vi "ISO-8601 UTC to Timestamp.vi"(11 "ISO-8601":string) -> (2 "error out":errorcluster, 3 "time stamp":timestamp)   [LabVIEW 2018, in "JSON.lvlib"]
uses:
  JSON.lvlib
  <vilib>/Utility/miscctls.llb/LVDateTimeRec.ctl
  <vilib>/regexp/Match Regular Expression.xnode
panel:
  out "whole match":string
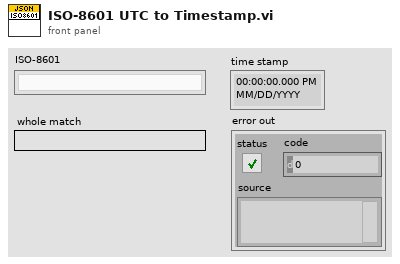
[diagram p1: front panel]
types:
  T1 = typedef "LVDateTimeRec.ctl" = cluster{"fractional second":dbl, "second":i32, "minute":i32, "hour":i32, "day of month":i32, "month":i32, "year":i32, "day of week":i32, "day of year":i32, "DST":i32}
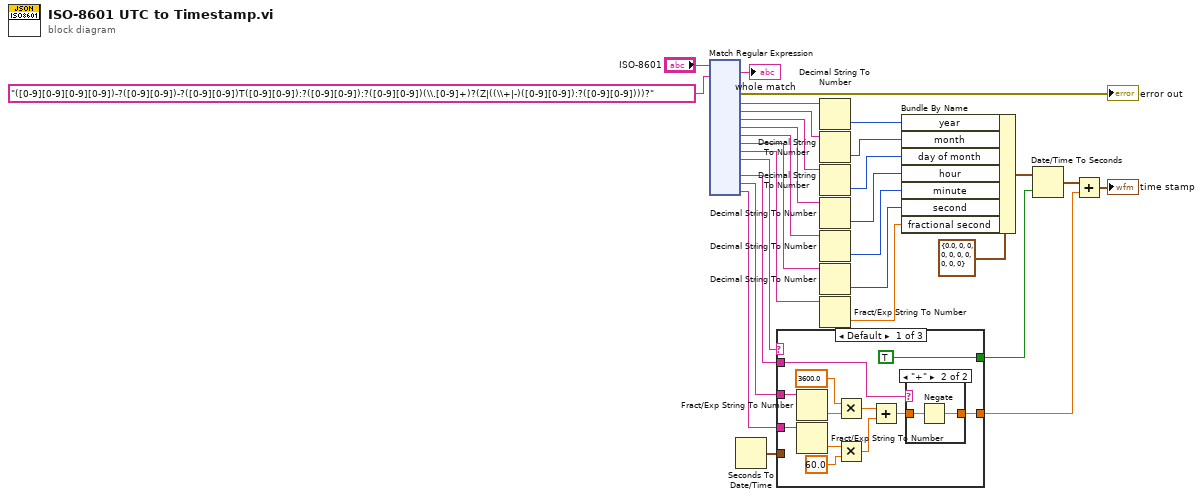
[diagram p0: block diagram]
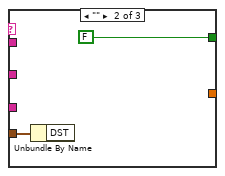
[diagram p3: hidden frame]
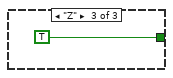
[diagram p4: hidden frame]
diagram:
  n1 = xnode "Match Regular Expression"("input string"="ISO-8601", "regular expression"="([0-9][0-9][0-9][0-9])-?([0-9][0-9])-?([0-9][0-9])T([0-9][0-9]):?([0-9][0-9]):?([0-9][0-9])(\\.[0-9]+)?(Z|((\\+|-)([0-9][0-9]):?([0-9][0-9])))?") -> ("whole match"=→"whole match":string, "error out"=→"error out":errorcluster, "submatch 1"=w27:string, "submatch 2"=w26:string, "submatch 3"=w17:string, "submatch 4"=w16:string, "submatch 5"=w15:string, "submatch 6"=w14:string, "submatch 7"=w13:string, "submatch 8"=w12:string, "submatch 10"=w11:string, "submatch 11"=w10:string, "submatch 12"=w9:string)  [unwired: 4 in, 4 out]
  n2 = Seconds To Date/Time() -> (date time rec=w2:T1)  [unwired: 2 in]
  n3 = case shown="Default" w12 {
    tunnel: w11 -> [w31 _ _]
    tunnel: w10 -> [w40 _ _]
    tunnel: w9 -> [w39 _ _]
    tunnel: [TRUE FALSE TRUE] -> w7
    tunnel: [w30 _ _] -> w4
    tunnel: w2 -> [_ w45 _]
    frame Default {
      n4 = Fract/Exp String To Number(string=w40) -> (number=w38:dbl)  [unwired: 3 in, 1 out]
      n5 = Fract/Exp String To Number(string=w39) -> (number=w37:dbl)  [unwired: 3 in, 1 out]
      n6 = Multiply(x=3600.0 ("y"), y=w38) -> (x*y=w34:dbl)
      n7 = Multiply(x=w37, y=60.0) -> (x*y=w33:dbl)
      n8 = Add(x=w34, y=w33) -> (x+y=w32:dbl)
      n9 = case shown="\"+\"" w31 {
        tunnel: w32 -> [w42 w44]
        tunnel: [w42 w43] -> w30
        frame Default {
        }
        frame "+" {
          n10 = Negate(x=w44) -> (-x=w43:dbl)
        }
      }
    }
    frame "" {
      n11 = Unbundle By Name(w45) -> ()  [unwired: 1 out]
    }
    frame "Z" {
    }
  }
  n12 = Decimal String To Number(string=w27) -> (number=w24:i32)  [unwired: 2 in, 1 out]
  n13 = Decimal String To Number(string=w26) -> (number=w23:i32)  [unwired: 2 in, 1 out]
  n14 = Decimal String To Number(string=w17) -> (number=w22:i32)  [unwired: 2 in, 1 out]
  n15 = Decimal String To Number(string=w16) -> (number=w21:i32)  [unwired: 2 in, 1 out]
  n16 = Decimal String To Number(string=w15) -> (number=w20:i32)  [unwired: 2 in, 1 out]
  n17 = Decimal String To Number(string=w14) -> (number=w19:i32)  [unwired: 2 in, 1 out]
  n18 = Fract/Exp String To Number(string=w13) -> (number=w18:dbl)  [unwired: 3 in, 1 out]
  n19 = Bundle By Name(cluster=T1 {"fractional second"=0.0, "second"=0, "minute"=0, "hour"=0, "day of month"=0, "month"=0, "year"=0, "day of week"=0, "day of year"=0, "DST"=0} ("date time rec"), "year"=w24, "month"=w23, "day of month"=w22, "hour"=w21, "minute"=w20, "second"=w19, "fractional second"=w18) -> (w8:T1)
  n20 = Date/Time To Seconds(1:w7, 2:w8) -> (0:w6:timestamp)
  n21 = Add(x=w6, y=w4) -> (x+y=→"time stamp":timestamp)
